vi "GT Get Di Reverse Count.vi"(6 "count":i16, 7 "pReverseCount":u32[](array[numeric]), 8 "error in (no error)":errorcluster caption="错误输入（无错误）", 9 "diIndex":i16, 10 "diType":i16, 11 "cardNum":i16) -> (0 "error out":errorcluster caption="错误输出", 3 "function return":i16, 5 "pReverseCount out":u32[](array[numeric]))   [LabVIEW 2014, in "gts.lvlib"]
doc: "GT_API GT_GetDiReverseCount(short cardNum,short diType,short diIndex,unsigned long *pReverseCount,short count=1);"
uses:
  gts.lvlib
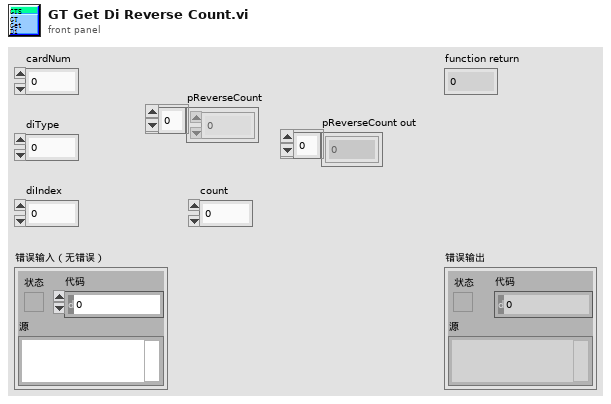
[diagram p1: front panel]
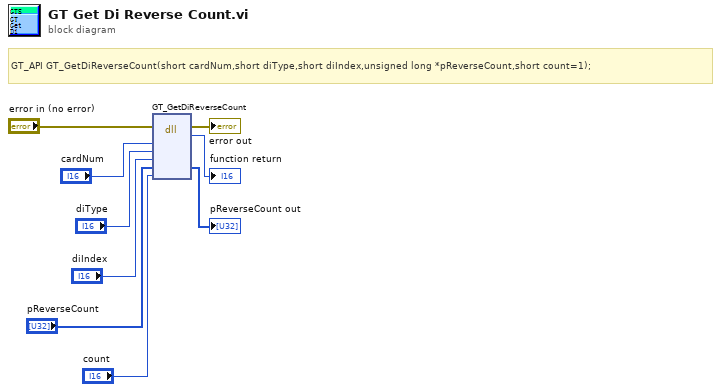
[diagram p0: block diagram]
diagram:
  # "GT_API GT_GetDiReverseCount(short cardNum,short diType,short diIndex,unsigned long *pReverseCount,short count=1);"
  n1 = dll-call lib="PTH2habs D固高科技资料GTS控制卡GTS卡18年上半年资料dllVC32bit\nmulti_cardgts.*" fn="GT_GetDiReverseCount"(error in="error in (no error)", "cardNum"="cardNum", "diType"="diType", "diIndex"="diIndex", "pReverseCount"="pReverseCount", "count"="count") -> (error out=→"error out":errorcluster, "返回类型"=→"function return":i16, "pReverseCount"=→"pReverseCount out":u32[])  [unwired: 6 in, 1 out]
